vi "Instr_SetPrivateData.vi"(8 "error in (no error)":errorcluster, 11 "WK6425 in":refnum<class "WK6425.lvclass">) -> (0 "error out":errorcluster, 3 "WK6425 out":refnum<class "WK6425.lvclass">)   [LabVIEW 2013, in "WK6425.lvclass"]
uses:
  WK6425.lvclass
  InstrumentSetup.vi
  WK6425_CommandsGlobal.vi
  InstrControl.lvclass
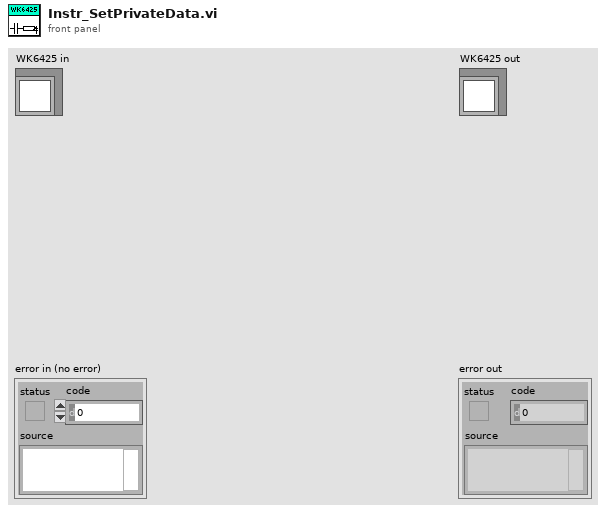
[diagram p1: front panel]
types:
  T1 = cluster{"RC Configuration":u16, "AC amplitude [V]":dbl, "AC frequency [Hz]":i32, "GPIB Address":string}
  T2 = cluster{"GPIB address":string, "Instrument name":string, "Instrument type":u16, "Command \"Initialise LCR\"":string, "Command \"OC Trim\"":string, "Command \"LCR Readout\"":string}
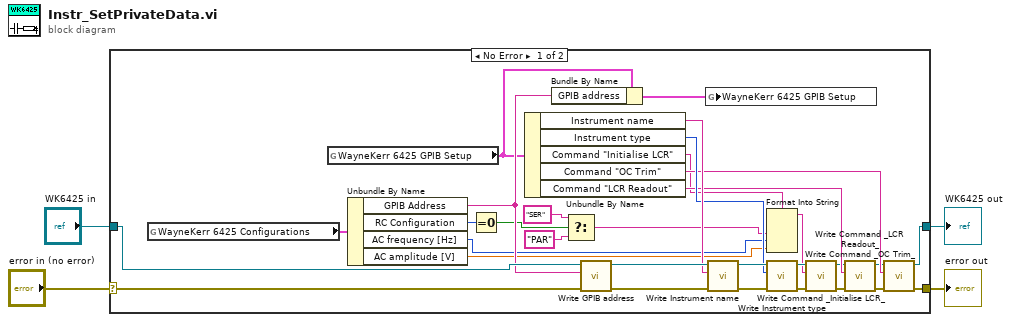
[diagram p0: block diagram]
diagram:
  n1 = case shown="No Error" "error in (no error)" {
    selector: "error in (no error)" -> [w30 w37]
    tunnel: [w19 w37] -> w3
    tunnel: [w20 w36] -> w4
    tunnel: "WK6425 in" -> [w35 w36]
    frame No Error {
      n2 = global read "InstrumentSetup.vi" "WayneKerr 6425 Configurations"() -> (w27:T1)
      n3 = global read "WK6425_CommandsGlobal.vi" "WayneKerr 6425 GPIB Setup"() -> (w6:T2)
      n4 = Unbundle By Name(w27) -> ("GPIB Address"=w26:string, "RC Configuration"=w15:u16, "AC frequency [Hz]"=w10:i32, "AC amplitude [V]"=w9:dbl)
      n5 = Equal To 0?(x=w15) -> (x = 0?=w14:bool)
      n6 = Unbundle By Name(w6) -> ("Instrument name"=w32:string, "Instrument type"=w31:u16, "Command \"Initialise LCR\""=w8:string, "Command \"OC Trim\""=w24:string, "Command \"LCR Readout\""=w25:string)
      n7 = Bundle By Name(cluster=w6, "GPIB address"=w26) -> (w5:T2)
      n8 = Select(t="SER", s=w14, f="PAR") -> (s? t:f=w11:string)
      n9 = call-dynamic "Write GPIB address.vi"("error in (no error)"=w30, "GPIB address"=w26, "InstControl in"=w35) -> ("error out"=w29:errorcluster, "InstControl out"=w34:refnum<class "WK6425.lvclass">)  [unwired: 7 in]
      n10 = global write "WK6425_CommandsGlobal.vi" "WayneKerr 6425 GPIB Setup"(w5) -> ()
      n11 = call-dynamic "Write Instrument name.vi"("error in (no error)"=w29, "Instrument name"=w32, "InstControl in"=w34) -> ("error out"=w28:errorcluster, "InstControl out"=w33:refnum<class "WK6425.lvclass">)  [unwired: 7 in]
      n12 = Format Into String(format string=w8, w11, w10, w9) -> (resulting string=w7:string)  [unwired: 2 in, 1 out]
      n13 = call-dynamic "Write Instrument type.vi"("error in (no error)"=w28, "Instrument type"=w31, "InstControl in"=w33) -> ("error out"=w16:errorcluster, "InstControl out"=w23:refnum<class "WK6425.lvclass">)  [unwired: 7 in]
      n14 = call-dynamic "Write Command _Initialise LCR_.vi"("error in (no error)"=w16, "Command \"Initialise LCR\""=w7, "LCRControl in"=w23) -> ("error out"=w18:errorcluster, "LCRControl out"=w22:refnum<class "WK6425.lvclass">)  [unwired: 7 in]
      n15 = call-dynamic "Write Command _LCR Readout_.vi"("error in (no error)"=w18, "Command \"LCR Readout\""=w25, "LCRControl in"=w22) -> ("error out"=w17:errorcluster, "LCRControl out"=w21:refnum<class "WK6425.lvclass">)  [unwired: 7 in]
      n16 = call-dynamic "Write Command _OC Trim_.vi"("error in (no error)"=w17, "Command \"OC Trim\""=w24, "LCRControl in"=w21) -> ("error out"=w19:errorcluster, "LCRControl out"=w20:refnum<class "WK6425.lvclass">)  [unwired: 7 in]
    }
    frame Error {
    }
  }
  "error out" <- w3
  "WK6425 out" <- w4
